vi "Actor Core.vi"(8 "error in":errorcluster, 11 "Nested in":refnum<class "Message Actor.lvclass">) -> (0 "error out":errorcluster, 3 "Actor out":refnum<class "Actor.lvclass">)   [LabVIEW 2020, in "Message Actor.lvlib" / "Message Actor.lvclass"]
doc: "(<B>Filename</B>: Actor Framework.lvlib:Actor.lvclass:Actor Core.vi)\n\nReceives messages to the actor, reacts to them, and initiates any error handling that may shut the actor down.\n\nDescendant classes may override this VI to append parallel tasks for the actor to complete while it handles messages. Overrides use the Call Parent Method node."
uses:
  Message Actor.lvclass
  C:/Program Files (x86)/National Instruments/LabVIEW 2020/vi.lib/ActorFramework/Actor/Actor.lvclass
  C:/Users/eddiews/Documents/Git Hub Repositorios/VendingMachine_ActorFramework/SubPanel Actor/SubPanel Actor/SubPanel Actor.lvclass
  <vilib>/ActorFramework/Actor/Actor.lvclass
  <vilib>/ActorFramework/Actor/Actor.lvclass/Actor.ctl
  <vilib>/ActorFramework/Message Enqueuer/Message Enqueuer.lvclass/Message Enqueuer.ctl
  Message Actor.lvclass/Message Actor.ctl
  SubPanel Actor/SubPanel Actor/SubPanel Actor.lvclass/SubPanel Actor.ctl
  Message Actor Messages/Send Message Msg/Send Message Msg.lvclass/Send Message Msg.ctl
  <vilib>/ActorFramework/Message Enqueuer/Init from Existing Queue.vi
  <vilib>/ActorFramework/Message Enqueuer/Enqueue.vi
  Message Actor Messages/Send Message Msg/Send Message Msg.lvclass
  C:/Program Files (x86)/National Instruments/LabVIEW 2020/vi.lib/ActorFramework/Message/Message.lvclass
  <vilib>/ActorFramework/Stop Msg/Stop Msg.lvclass
  <vilib>/ActorFramework/Message Priority Queue/Priority Enqueue.vi
  <vilib>/ActorFramework/Message Enqueuer/Message Enqueuer.lvclass
  SubPanel Actor/SubPanel Actor/SubPanel Actor.lvclass
  C:/Users/eddiews/Documents/Git Hub Repositorios/VendingMachine_ActorFramework/Message Actor/Message Actor.lvclass
panel:
  out "Messaje String":string
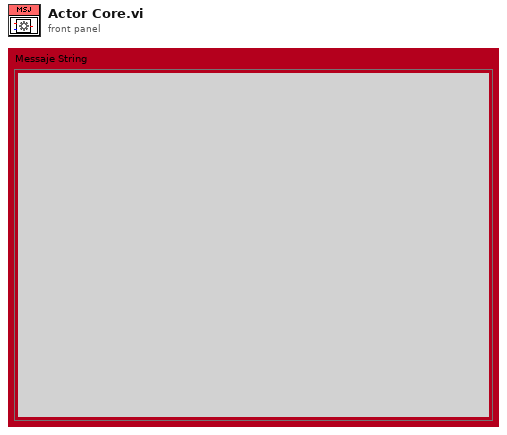
[diagram p1: front panel]
types:
  T1 = cluster{"Stop":refnum<user-event>, "Messaje String":refnum<user-event>}
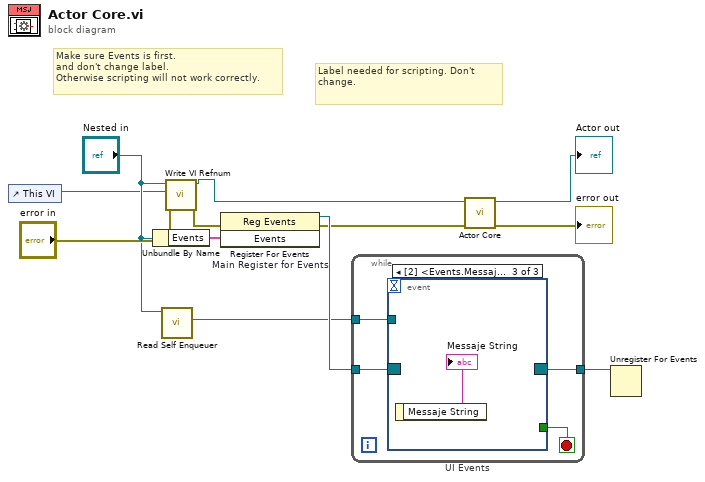
[diagram p0: block diagram]
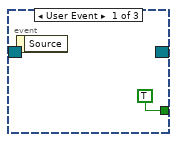
[diagram p2: hidden frame]
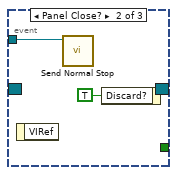
[diagram p3: hidden frame]
diagram:
  # "Label needed for scripting. Don't change."
  # "Make sure Events is first.\nand don't change label.\nOtherwise scripting will not work correctly."
  n1 = control-ref of="This VI"() -> (w2:refnum<vi>)
  n2 = Unbundle By Name("Nested in") -> ("Events"=w9:T1)
  n3 = call <vilib>:"Read Self Enqueuer.vi"("Actor"="Nested in") -> ("Self Enqueuer"=w7:refnum<class "Message Enqueuer.lvclass">)  [unwired: 10 in]
  n4 = call "Write VI Refnum.vi"("error in (no error)"="error in", "VI Refnum"=w2, "SubPanel Actor in"="Nested in") -> ("error out"=w5:errorcluster, "SubPanel Actor out"=w1:refnum<class "Message Actor.lvclass">)  [unwired: 7 in]
  n5 = register-events "Main Register for Events"(error in=w5, w9) -> (reference out=w10:refnum<event-registration>, error out=w6:errorcluster)  [unwired: 1 in]
  n6 = while {
    tunnel: w10 -> [w16]
    tunnel: [w14] -> w8
    tunnel: w7 -> [w13]
    stop <- w15 stop-if-true
    n7 = event "UI Events" shown="[2] <Events.Messaje String>: User Event" {
      selector: w16 -> [_ _ _]
      dyn-events: [_ _ _] -> w14
      timeout: _ -> [_ _ _]
      tunnel: [TRUE _ _] -> w15
      tunnel: w13 -> [_ w18 _]
      event User Event {
        n8 = event-data() -> ()  [unwired: 1 in, 1 out]
      }
      event Panel Close? {
        n9 = event-data() -> ()  [unwired: 1 in, 1 out]
        n10 = call <vilib>:"Send Normal Stop.vi"("Message Enqueuer"=w18) -> ()  [unwired: 10 in, 1 out]
        n11 = event-data("Discard?"=TRUE) -> ()  [unwired: 1 in, 1 out]
      }
      event User Event {
        n12 = event-data() -> ("Messaje String"=→"Messaje String":string)  [unwired: 1 in]
      }
    }
  }
  n13 = call-parent "Actor Core.vi"("error in"=w6, "Actor in"=w1) -> ("error out"=→"error out":errorcluster, "Actor out"=→"Actor out":refnum<class "Actor.lvclass">)  [unwired: 8 in]
  n14 = Unregister For Events(event registration refnum=w8) -> ()  [unwired: 1 in, 1 out]
